vi "Write_Logfile.vi"(1 "path":path, 2 "System Monitor Variables (in)":T1) -> ()   [LabVIEW 2016]
uses:
  Global/Global Variables/System Monitor Cluster.ctl
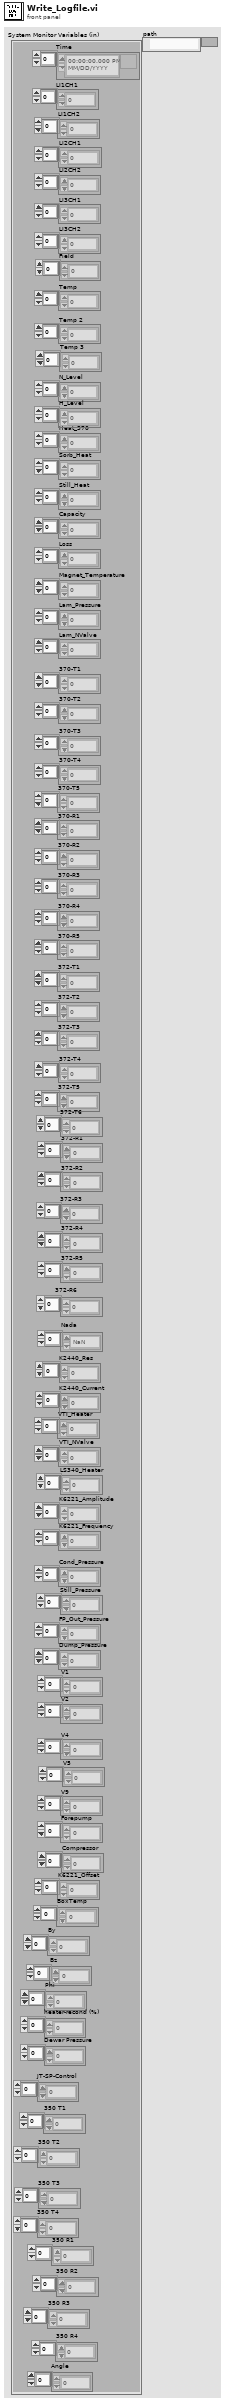
[diagram p1: front panel]
types:
  T1 = typedef "System Monitor Cluster.ctl" = cluster{"Time":timestamp[], "LI1CH1":dbl[], "LI1CH2":dbl[], "LI2CH1":dbl[], "LI2CH2":dbl[], "LI3CH1":dbl[], "LI3CH2":dbl[], "Field":dbl[], "Temp":dbl[], "Temp 2":dbl[], "Temp 3":dbl[], "N_Level":dbl[], "H_Level":dbl[], "Heat_370":dbl[], "Sorb_Heat":dbl[], "Still_Heat":dbl[], "Capacity":dbl[], "Loss":dbl[], "Magnet_Temperature":dbl[], "Lam_Pressure":dbl[], "Lam_NValve":dbl[], "370-T1":dbl[], "370-T2":dbl[], "370-T3":dbl[], "370-T4":dbl[], "370-T5":dbl[], "370-R1":dbl[], "370-R2":dbl[], "370-R3":dbl[], "370-R4":dbl[], "370-R5":dbl[], "372-T1":dbl[], "372-T2":dbl[], "372-T3":dbl[], "372-T4":dbl[], "372-T5":dbl[], "372-T6":dbl[], "372-R1":dbl[], "372-R2":dbl[], "372-R3":dbl[], "372-R4":dbl[], "372-R5":dbl[], "372-R6":dbl[], "Nada":dbl[], "K2440_Res":dbl[], "K2440_Current":dbl[], "VTI_Heater":dbl[], "VTI_NValve":dbl[], "LS340_Heater":dbl[], "K6221_Amplitude":dbl[], "K6221_Frequency":dbl[], "Cond_Pressure":dbl[], "Still_Pressure":dbl[], "FP_Out_Pressure":dbl[], "Dump_Pressure":dbl[], "V1":dbl[], "V2":dbl[], "V4":dbl[], "V5":dbl[], "V9":dbl[], "Forepump":dbl[], "Compressor":dbl[], "K6221_Offset":dbl[], "BoxTemp":dbl[], "By":dbl[], "Bz":dbl[], "Phi":dbl[], "heater-recond (%)":dbl[], "Dewar Pressure ":dbl[], "JT-SP-Control":dbl[], "350 T1":dbl[], "350 T2":dbl[], "350 T3":dbl[], "350 T4":dbl[], "350 R1":dbl[], "350 R2":dbl[], "350 R3":dbl[], "350 R4":dbl[], "Angle":dbl[]}
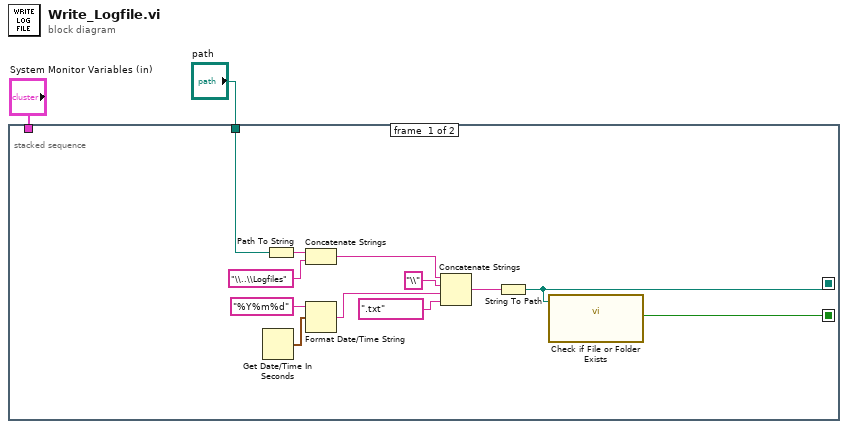
[diagram p0: block diagram]
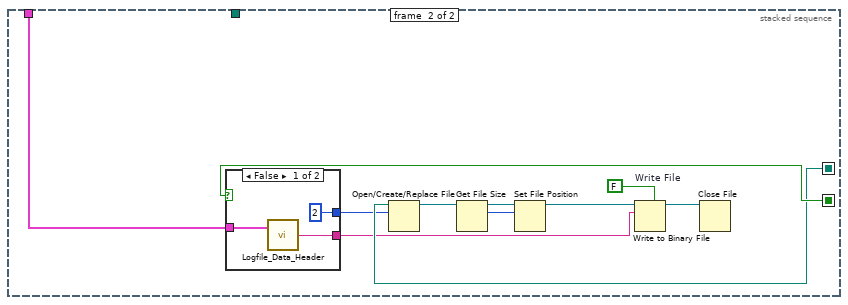
[diagram p2: hidden frame]
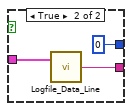
[diagram p3: hidden frame]
diagram:
  n1 = stacked-sequence {
    seq-local: [w8 _] -> [_ w25]
    seq-local: [w7 _] -> [_ w24]
    tunnel: "System Monitor Variables (in)" -> [_ w15]
    tunnel: "path" -> [w3 _]
    frame #0 {
      n2 = Get Date/Time In Seconds() -> (seconds since 1Jan1904=w13:timestamp)
      n3 = Path To String(path=w3) -> (string=w6:string)
      n4 = Concatenate Strings(w6, "\\..\\Logfiles") -> (w4:string)
      n5 = Format Date/Time String(time format string (%c)="%Y%m%d", seconds (now)=w13) -> (date/time string=w12:string)  [unwired: 1 in]
      n6 = Concatenate Strings(w4, "\\", w12, ".txt") -> (w9:string)
      n7 = String To Path(string=w9) -> (path=w7:path)
      n8 = call <vilib>:"Check if File or Folder Exists.vi"("path"=w7) -> ("file or folder exists?"=w8:bool)  [unwired: 8 in, 2 out]
    }
    frame #1 {
      n9 = case shown="False" w25 {
        tunnel: [w27 w31] -> w22
        tunnel: w15 -> [w26 w30]
        tunnel: [2 0] -> w23
        frame False {
          n10 = call "Logfile_Data_Header.vi"("System Monitor Cluster"=w26) -> ("Data Line"=w27:string)  [unwired: 1 in]
        }
        frame True {
          n11 = call "Logfile_Data_Line.vi"("System Monitor Cluster"=w30) -> ("Data Line"=w31:string)  [unwired: 1 in]
        }
      }
      n12 = Open/Create/Replace File(file path (use dialog)=w24, operation (0:open)=w23) -> (refnum out=w18:refnum<file>)  [unwired: 4 in, 2 out]
      n13 = Get File Size(file=w18) -> (refnum out=w17:refnum<file>, size (in bytes)=w16:i64)  [unwired: 1 in, 1 out]
      n14 = Set File Position(offset (in bytes) (0)=w16, refnum=w17) -> (refnum out=w19:refnum<file>)  [unwired: 2 in, 1 out]
      n15 = Write to Binary File "Write File"(file (use dialog)=w19, data=w22, 5:FALSE) -> (refnum out=w21:refnum<file>)  [unwired: 3 in, 2 out]
      n16 = Close File(refnum=w21) -> ()  [unwired: 1 in, 2 out]
    }
  }
